vi "Flush Toveys.vi"(8 "error in (no error)":errorcluster, 11 "Model in":refnum<class "Model.lvclass">) -> (0 "error out":errorcluster, 3 "Model out":refnum<class "Model.lvclass">)   [LabVIEW 2016]
uses:
  TEI-9150/Tovey 9150.lvclass
  Model.lvclass
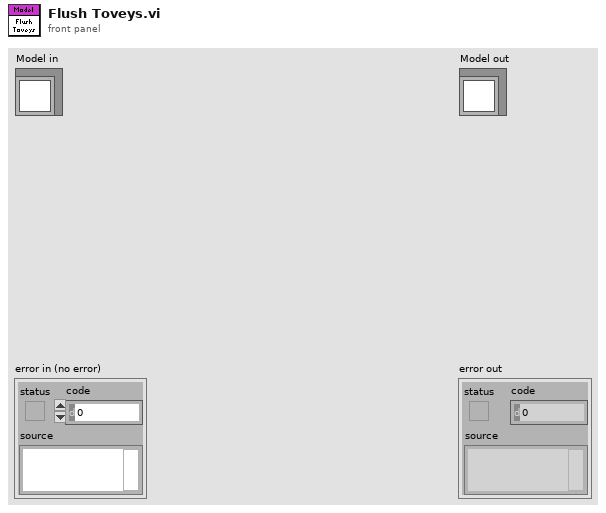
[diagram p1: front panel]
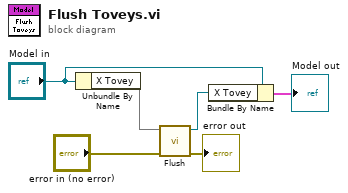
[diagram p0: block diagram]
diagram:
  n1 = Unbundle By Name("Model in") -> ("X Tovey"=w4)
  n2 = call "Flush.vi"("error in (no error)"="error in (no error)", "Tovey 9150 in"=w4) -> ("error out"=→"error out":errorcluster, "Tovey 9150 out"=w3:refnum<class "Tovey 9150.lvclass">)  [unwired: 8 in]
  n3 = Bundle By Name(cluster="Model in", "X Tovey"=w3) -> (→"Model out":cluster{})
